vi "Configure Tasks And Channels.vi"(11 "DAQmx Shortcuts":T1[](array[typedef])) -> (2 "Task Per Device":refnum<k21>[](array[refnum]), 3 "DAQmx Shortcuts Per Device":cluster{T1[]}[](array[cluster]))   [LabVIEW 2019, in "DAQmx.lvlib"]
doc: "Map channels to devices, creating one task per device with those channels. Output is a jagged 2D array of devices & channels, where there could be 1-n channels per device."
uses:
  DAQmx.lvlib
  DAQmx Shortcut.ctl
  <vilib>/DAQmx/configure/timing.llb/DAQmx Timing (Sample Clock).vi
  <resource>/objmgr/daqmx.rc
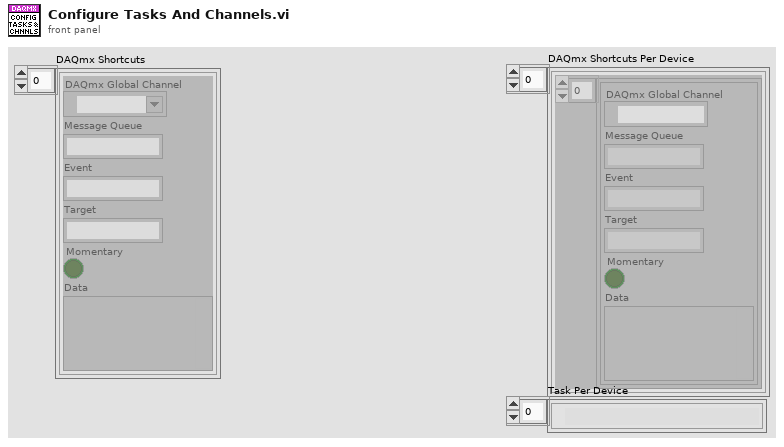
[diagram p1: front panel]
types:
  T1 = typedef "DAQmx.lvlib/DAQmx Shortcut.ctl" = cluster{"DAQmx Global Channel":refnum<k21>, "Message Queue":string, "Event":string, "Target":string, "Momentary":bool, "Data":variant}
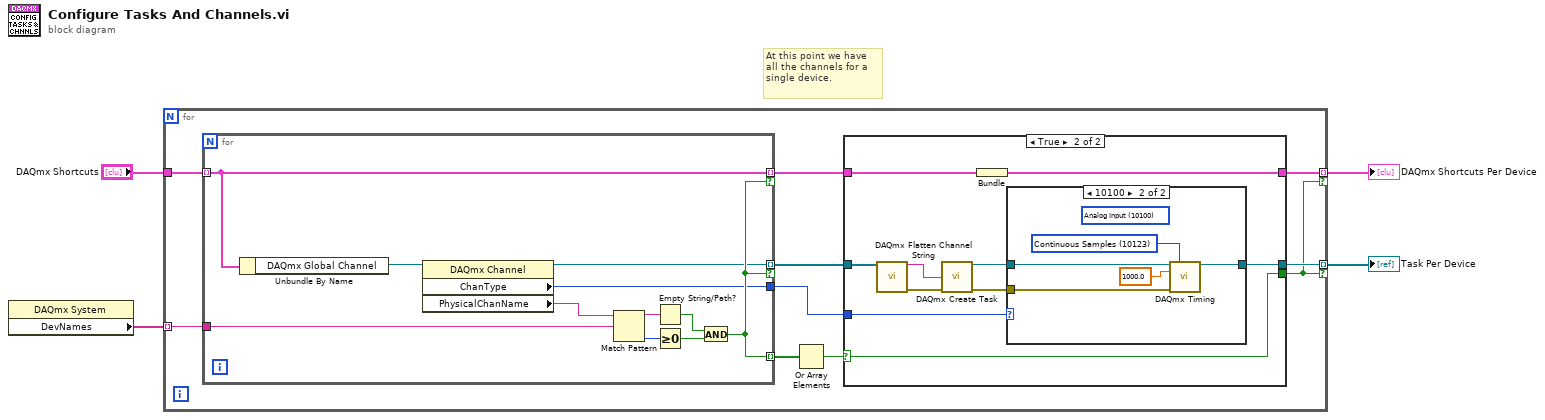
[diagram p0: block diagram]
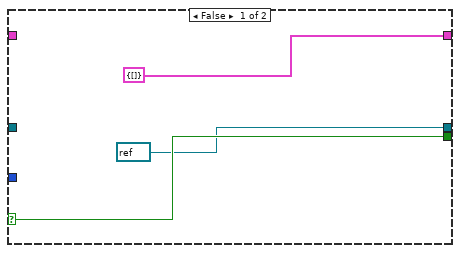
[diagram p2: hidden frame]
diagram:
  # "At this point we have all the channels for a single device."
  n1 = property class="DAQmx System"() -> ("DevNames"=w4:tag[])  [unwired: 2 in, 2 out]
  n2 = for {
    tunnel: w4 -> [w14] mode=indexing
    tunnel: [w10] -> w1 mode=indexing if=w8
    tunnel: "DAQmx Shortcuts" -> [w9]
    tunnel: [w6] -> w2 mode=indexing if=w8
    n3 = for {
      tunnel: w14 -> [w44]
      tunnel: [w39] -> w13 mode=indexing
      tunnel: [w37] -> w11 mode=indexing if=w39
      tunnel: w9 -> [w36] mode=indexing
      tunnel: [w36] -> w7 mode=indexing if=w39
      tunnel: [w34] -> w5
      n4 = Unbundle By Name(w36) -> ("DAQmx Global Channel"=w35:refnum<k21>)
      n5 = property class="DAQmx Channel"(reference=w35) -> (reference out=w37:refnum<k21>, "ChanType"=w34:i32, "PhysicalChanName"=w38:tag)  [unwired: 1 in, 1 out]
      n6 = Match Pattern(string=w38, regular expression=w44) -> (before substring=w43:string, offset past match=w42:i32)  [unwired: 1 in, 2 out]
      n7 = Empty String/Path?(string/path=w43) -> (empty?=w41:bool)
      n8 = Greater Or Equal To 0?(x=w42) -> (x >= 0?=w40:bool)
      n9 = And(x=w41, y=w40) -> (x .and. y?=w39:bool)
    }
    n10 = Or Array Elements(Boolean array=w13) -> (logical OR=w12:bool)
    n11 = case shown="True" w12 {
      selector: w12 -> [w17 w22]
      tunnel: w11 -> [_ w21]
      tunnel: [refnum<k21> refnum ("task out") w23] -> w10
      tunnel: [w17 w22] -> w8
      tunnel: w7 -> [_ w20]
      tunnel: [cluster{T1[]} {[]} w19] -> w6
      tunnel: w5 -> [_ w18]
      frame False {
      }
      frame True {
        n12 = call <vilib>:"DAQmx Flatten Channel String.vi"("names in"=w21) -> ("names out"=w25:string, "error out"=w24:errorcluster)  [unwired: 13 in]
        n13 = call <vilib>:"DAQmx Create Task.vi"("global virtual channels"=w25, "error in"=w24) -> ("task out"=w27:refnum<k21>, "error out"=w26:errorcluster)  [unwired: 12 in]
        n14 = Bundle(w20) -> (w19:cluster{T1[]})  [unwired: 1 in]
        n15 = case shown="10100" w18 {
          tunnel: w27 -> [w28 w31]
          tunnel: w26 -> [_ w30]
          tunnel: [w28 w29] -> w23
          frame Default {
          }
          frame 10100 {
            (unwired) 10100 items=["Analog Input"=10100, "Analog Output"=10102, "Digital Input"=10151, "Digital Output"=10153, "Counter Input"=10131, "Counter Output"=10132] ("ChanType")
            w32 = 10123 items=["Finite Samples"=10178, "Continuous Samples"=10123, "Hardware Timed Single Point"=12522] ("sample mode")
            n16 = call-poly <vilib>:"DAQmx Timing.vi"("task/channels in"=w31, "sample mode"=w32, "rate"=1000.0, "error in"=w30) -> ("task out"=w29:refnum<k21>)  [unwired: 10 in, 1 out]
          }
        }
      }
    }
  }
  "DAQmx Shortcuts Per Device" <- w2
  "Task Per Device" <- w1
